vi "Agilent Start Button.vi"(0 "Station In":string, 1 "Agilent Channels In":T2[](array[typedef])=[{"Channel"="301", "Station"="1", "Label"="Water Valve", "Agilent Station"="2"}, {"Channel"="302", "Station"="2", "Label"="Water Valve", "Agilent Station"="2"}, {"Channel"="303", "Station"="3", "Label"="Water Valve", "Agilent Station"="2"}, {"Channel"="304", "Station"="4", "Label"="Water Valve", "Agilent Station"="2"}, {"Channel"="305", "Station"="5", "Label"="Water Valve", "Agilent Station"="2"}, {"Channel"="306", "Station"="6", "Label"="Water Valve", "Agilent Station"="2"}, {"Channel"="307", "Station"="7", "Label"="Water Valve", "Agilent Station"="2"}, {"Channel"="308", "Station"="8", "Label"="Water Valve", "Agilent Station"="2"}, {"Channel"="309", "Station"="9", "Label"="Water Valve", "Agilent Station"="2"}, {"Channel"="310", "Station"="10", "Label"="Water Valve", "Agilent Station"="2"}, {"Channel"="311", "Station"="11", "Label"="Water Valve", "Agilent Station"="2"}, {"Channel"="312", "Station"="12", "Label"="Water Valve", "Agilent Station"="2"}, {"Channel"="313", "Station"="13", "Label"="Water Valve", "Agilent Station"="2"}, {"Channel"="314", "Station"="14", "Label"="Water Valve", "Agilent Station"="2"}, {"Channel"="315", "Station"="15", "Label"="Water Valve", "Agilent Station"="2"}, {"Channel"="316", "Station"="16", "Label"="Water Valve", "Agilent Station"="2"}, {"Channel"="317", "Station"="17", "Label"="Water Valve", "Agilent Station"="2"}, {"Channel"="318", "Station"="18", "Label"="Water Valve", "Agilent Station"="2"}, {"Channel"="319", "Station"="19", "Label"="Water Valve", "Agilent Station"="2"}, {"Channel"="320", "Station"="20", "Label"="Water Valve", "Agilent Station"="2"}, {"Channel"="101", "Station"="21", "Label"="Water Valve", "Agilent Station"="3"}, {"Channel"="102", "Station"="22", "Label"="Water Valve", "Agilent Station"="3"}, {"Channel"="103", "Station"="23", "Label"="Water Valve", "Agilent Station"="3"}, {"Channel"="104", "Station"="24", "Label"="Water Valve", "Agilent Station"="3"}, {"Channel"="105", "Station"="25", "Label"="Water Valve", "Agilent Station"="3"}, {"Channel"="106", "Station"="26", "Label"="Water Valve", "Agilent Station"="3"}, {"Channel"="107", "Station"="27", "Label"="Water Valve", "Agilent Station"="3"}, {"Channel"="108", "Station"="28", "Label"="Water Valve", "Agilent Station"="3"}, {"Channel"="109", "Station"="29", "Label"="Water Valve", "Agilent Station"="3"}, {"Channel"="110", "Station"="30", "Label"="Water Valve", "Agilent Station"="3"}, {"Channel"="111", "Station"="31", "Label"="Water Valve", "Agilent Station"="3"}, {"Channel"="112", "Station"="32", "Label"="Water Valve", "Agilent Station"="3"}, {"Channel"="101", "Station"="33", "Label"="Water Valve", "Agilent Station"="5"}, {"Channel"="102", "Station"="34", "Label"="Water Valve", "Agilent Station"="5"}, {"Channel"="103", "Station"="35", "Label"="Water Valve", "Agilent Station"="5"}, {"Channel"="104", "Station"="36", "Label"="Water Valve", "Agilent Station"="5"}, {"Channel"="105", "Station"="37", "Label"="Water Valve", "Agilent Station"="5"}, {"Channel"="106", "Station"="38", "Label"="Water Valve", "Agilent Station"="5"}, {"Channel"="107", "Station"="39", "Label"="Water Valve", "Agilent Station"="5"}, {"Channel"="108", "Station"="40", "Label"="Water Valve", "Agilent Station"="5"}, {"Channel"="109", "Station"="41", "Label"="Water Valve", "Agilent Station"="5"}, {"Channel"="110", "Station"="42", "Label"="Water Valve", "Agilent Station"="5"}, {"Channel"="111", "Station"="43", "Label"="Water Valve", "Agilent Station"="5"}, {"Channel"="112", "Station"="44", "Label"="Water Valve", "Agilent Station"="5"}, {"Channel"="113", "Station"="45", "Label"="Water Valve", "Agilent Station"="5"}, {"Channel"="114", "Station"="46", "Label"="Water Valve", "Agilent Station"="5"}, {"Channel"="115", "Station"="47", "Label"="Water Valve", "Agilent Station"="5"}, {"Channel"="116", "Station"="48", "Label"="Water Valve", "Agilent Station"="5"}, {"Channel"="117", "Station"="49", "Label"="Water Valve", "Agilent Station"="5"}, {"Channel"="118", "Station"="50", "Label"="Water Valve", "Agilent Station"="5"}, {"Channel"="119", "Station"="51", "Label"="Water Valve", "Agilent Station"="5"}, {"Channel"="120", "Station"="52", "Label"="Water Valve", "Agilent Station"="5"}, {"Channel"="201", "Station"="53", "Label"="Water Valve", "Agilent Station"="5"}, {"Channel"="202", "Station"="54", "Label"="Water Valve", "Agilent Station"="5"}, {"Channel"="203", "Station"="55", "Label"="Water Valve", "Agilent Station"="5"}, {"Channel"="204", "Station"="56", "Label"="Water Valve", "Agilent Station"="5"}], 2 "Agilent":T1, 5 "Open/Close (F:Close)":bool, 11 "error in (no error)":errorcluster) -> (6 "Success":bool, 15 "error out":errorcluster)   [LabVIEW 2012]
uses:
  Agilent Channel Definition.ctl
  Drivers/Agilent 34970/Agilent 34970.lvlib
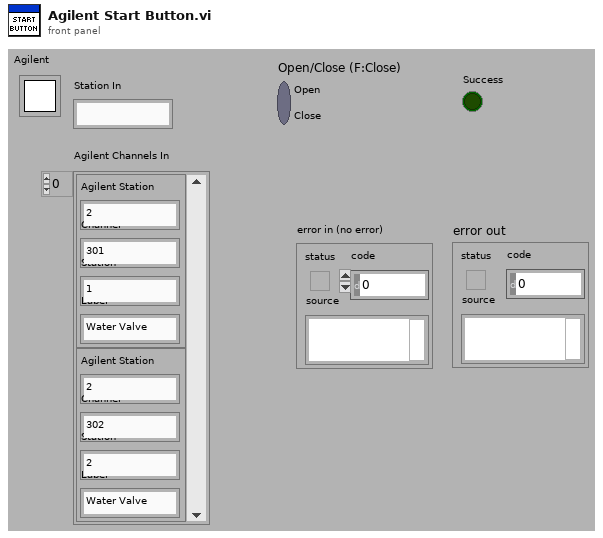
[diagram p1: front panel]
types:
  T1 = typedef "Semaphore RefNum" = refnum<k1>
  T2 = typedef "Agilent Channel Definition.ctl" = cluster{"Channel":string, "Station":string, "Label":string, "Agilent Station":string}
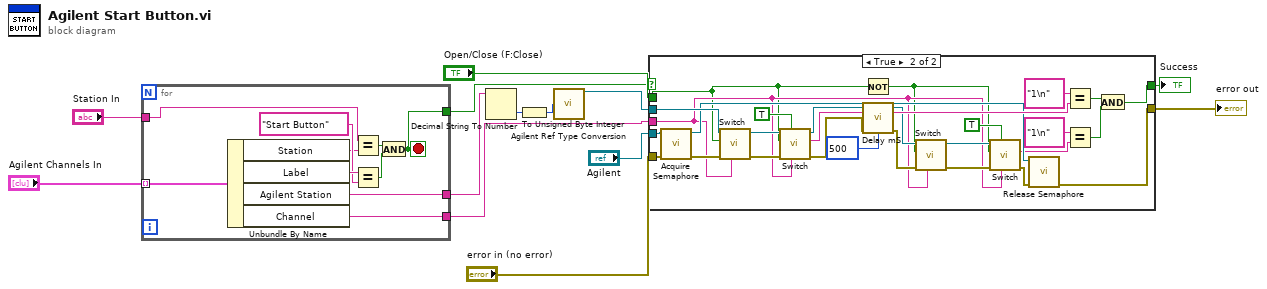
[diagram p0: block diagram]
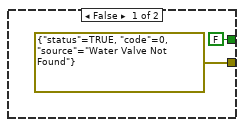
[diagram p2: hidden frame]
diagram:
  n1 = for {
    tunnel: "Agilent Channels In" -> [w23] mode=indexing
    tunnel: "Station In" -> [w18]
    tunnel: [w16] -> w12
    tunnel: [w15] -> w5
    tunnel: [w14] -> w4
    stop <- w14 stop-if-true
    n2 = Unbundle By Name(w23) -> ("Station"=w19:string, "Label"=w22:string, "Agilent Station"=w16:string, "Channel"=w15:string)
    n3 = Equal?(x=w18, y=w19) -> (x = y?=w17:bool)
    n4 = Equal?(x=w22, y="Start Button") -> (x = y?=w20:bool)
    n5 = And(x=w17, y=w20) -> (x .and. y?=w14:bool)
  }
  n6 = Decimal String To Number(string=w12) -> (number=w11:i32)  [unwired: 2 in, 1 out]
  n7 = To Unsigned Byte Integer(number=w11) -> (unsigned 8bit integer=w10:u8)
  n8 = call "Agilent Ref Type Conversion.vi"("Agilent Ref"=w10) -> ("VISA resource name"=w9:refnum<visa-resource-name>)  [unwired: 14 in]
  n9 = case shown="True" w4 {
    tunnel: w9 -> [_ w52]
    tunnel: "Open/Close (F:Close)" -> [_ w27]
    tunnel: "error in (no error)" -> [_ w45]
    tunnel: [errorcluster {"status"=TRUE, "code"=0, "source"="Water Valve Not Found"} ("error out") w43] -> w6
    tunnel: w5 -> [_ w29]
    tunnel: [FALSE w31] -> w3
    tunnel: "Agilent" -> [_ w46]
    frame False {
    }
    frame True {
      n10 = call <vilib>:"Acquire Semaphore.vi"("error in (no error)"=w45, "semaphore"=w46) -> ("error out"=w44:errorcluster, "semaphore out"=w42:T1)  [unwired: 3 in, 1 out]
      n11 = call "Switch.vi"("Channel List(empty)"=w29, "error in (no error)"=w44, "Open/Close (F:Close)"=w27, "VISA Resource Name"=w52) -> ("error out"=w51:errorcluster, "VISA Resource Name Out"=w50:refnum<visa-resource-name>)  [unwired: 5 in, 1 out]
      n12 = call "Switch.vi"("Channel List(empty)"=w29, "Set/Check (F:Set)"=TRUE, "error in (no error)"=w51, "Open/Close (F:Close)"=w27, "VISA Resource Name"=w50) -> ("error out"=w41:errorcluster, "Channel State?"=w48:string, "VISA Resource Name Out"=w36:refnum<visa-resource-name>)  [unwired: 4 in]
      n13 = Not(x=w27) -> (.not. x?=w26:bool)
      n14 = call "Delay mS.vi"("Error In"=w41, "milliseconds to wait"=u32 500) -> ("Error Out"=w38:errorcluster)  [unwired: 13 in]
      n15 = call "Switch.vi"("Channel List(empty)"=w29, "error in (no error)"=w38, "Open/Close (F:Close)"=w26, "VISA Resource Name"=w36) -> ("error out"=w39:errorcluster, "VISA Resource Name Out"=w35:refnum<visa-resource-name>)  [unwired: 5 in, 1 out]
      n16 = call "Switch.vi"("Channel List(empty)"=w29, "Set/Check (F:Set)"=TRUE, "error in (no error)"=w39, "Open/Close (F:Close)"=w26, "VISA Resource Name"=w35) -> ("error out"=w37:errorcluster, "Channel State?"=w32:string)  [unwired: 4 in, 1 out]
      n17 = call <vilib>:"Release Semaphore.vi"("error in (no error)"=w37, "semaphore"=w42) -> ("error out"=w43:errorcluster)  [unwired: 4 in, 1 out]
      n18 = Equal?(x="1\n" ("Channel State?"), y=w48) -> (x = y?=w28:bool)
      n19 = Equal?(x="1\n" ("Channel State?"), y=w32) -> (x = y?=w30:bool)
      n20 = And(x=w28, y=w30) -> (x .and. y?=w31:bool)
    }
  }
  "error out" <- w6
  "Success" <- w3
